vi "Checksum.vi"(3 "string to write":string="*IDN?") -> (1 "ASCII Output":string)   [LabVIEW 2013]
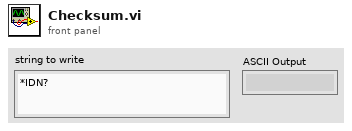
[diagram p1: front panel]
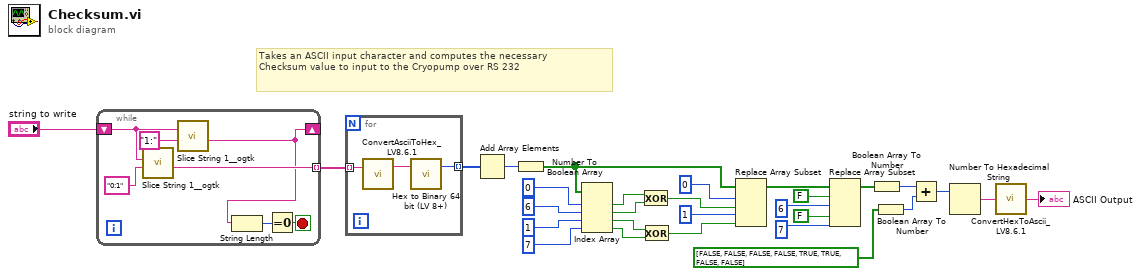
[diagram p0: block diagram]
diagram:
  # "Takes an ASCII input character and computes the necessary\nChecksum value to input to the Cryopump over RS 232"
  n1 = while {
    tunnel: [w31] -> w1 mode=indexing
    shift-right: [w30] -> _
    shift-left: "string to write" -> [w32]
    stop <- w35 stop-if-true
    n2 = call <userlib>:"Slice String 1__ogtk.vi"("Subset (i:j)"="0:1", "String"=w32) -> ("Substring (String[i:j])"=w31:string)  [unwired: 7 in]
    n3 = call <userlib>:"Slice String 1__ogtk.vi"("Subset (i:j)"="1:", "String"=w32) -> ("Substring (String[i:j])"=w30:string)  [unwired: 7 in]
    n4 = String Length(string=w30) -> (length=w36:i32)
    n5 = Equal To 0?(x=w36) -> (x = 0?=w35:bool)
  }
  n6 = for {
    tunnel: [w38] -> w4 mode=indexing
    tunnel: w1 -> [w37] mode=indexing
    n7 = call "ConvertAsciiToHex_LV8.6.1.vi"("ASCII Input String"=w37) -> ("Hexadecimal Output"=w39:string)  [unwired: 2 in]
    n8 = call "Hex to Binary 64 bit (LV 8+).vi"("Hexadecimal String"=w39) -> ("unsigned 8bit integer"=w38:u8)  [unwired: 2 in]
  }
  n9 = Add Array Elements(numeric array=w4) -> (sum=w3:u8)
  n10 = Number To Boolean Array(number=w3) -> (Boolean array=w9:bool[])
  n11 = Index Array(array=w9, index #1=0 ("index"), index #2=6 ("index"), index #3=1 ("index"), index #4=7 ("index")) -> (element #1=w25:bool, element #2=w24:bool, element #3=w23:bool, element #4=w22:bool)
  n12 = Exclusive Or(1:w24, 2:w25) -> (0:w16:bool)
  n13 = Exclusive Or(1:w22, 2:w23) -> (0:w14:bool)
  n14 = Replace Array Subset(array=w9, new element #1=w16, index #1=0 ("index"), new element #2=w14, index #2=1 ("index")) -> (w13:bool[])
  n15 = Replace Array Subset(array=w13, new element #1=FALSE ("new element/subarray"), index #1=6 ("index"), new element #2=FALSE ("new element/subarray"), index #2=7 ("index")) -> (w7:bool[])
  n16 = Boolean Array To Number(Boolean array=w7) -> (number=w12:u32)
  n17 = Boolean Array To Number(Boolean array=bool[] [FALSE, FALSE, FALSE, FALSE, TRUE, TRUE, FALSE, FALSE] ("y")) -> (number=w5:u32)
  n18 = Add(x=w12, y=w5) -> (x+y=w6:u32)
  n19 = Number To Hexadecimal String(2:w6) -> (0:w11:string)  [unwired: 1 in]
  n20 = call "ConvertHexToAscii_LV8.6.1.vi"("Hexadecimal Input String"=w11) -> ("ASCII Output"=→"ASCII Output":string)
